vi "TouchMux-API.vi"(11 "Connection":u8) -> (0 "t3":bool, 1 "t2":bool, 2 "t1":bool, 3 "Result Value":i16)   [LabVIEW 2010]
uses:
  mindsensors-library.llb/NXTInputRefnum.ctl
  <vilib>/NXT/Block Support/HWPage.SensorType.ctl
  <vilib>/NXT/Block Support/HWPage.SensorMode.ctl
  resource/objmgr/NXTInputOutput.rc
panel:
  in  "H123":u16=800
  in  "L123":u16=724
  in  "H23":u16=723
  in  "L23":u16=659
  in  "H13":u16=658
  in  "L13":u16=600
  in  "H3":u16=599
  in  "L3":u16=500
  in  "H12":u16=460
  in  "L12":u16=370
  in  "H2":u16=290
  in  "L2":u16=210
  in  "H1":u16=160
  in  "L1":u16=60
  in  "Generic Refnum Name":T1
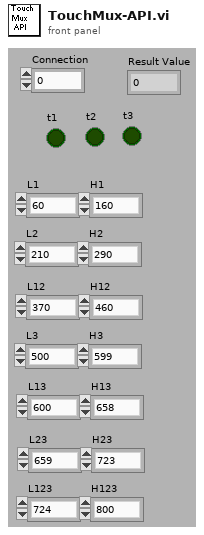
[diagram p1: front panel]
types:
  T1 = typedef "NXTInputRefnum.ctl" = refnum<k21>
  T2 = typedef "HWPage.SensorType.ctl" = u8
  T3 = typedef "HWPage.SensorMode.ctl" = u8
  T4 = typedef "NXT_InputPort.ctl" = u8
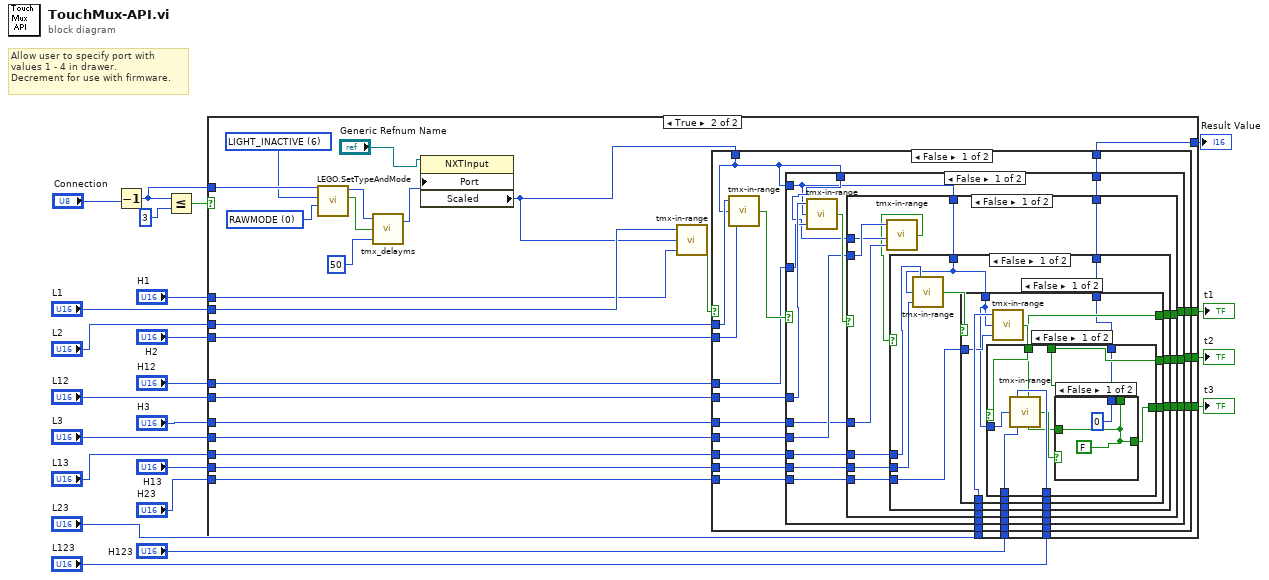
[diagram p0: block diagram]
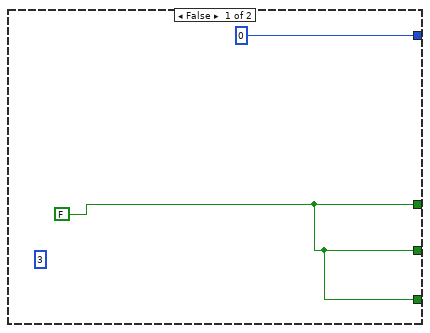
[diagram p2: hidden frame]
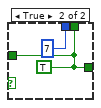
[diagram p3: hidden frame]
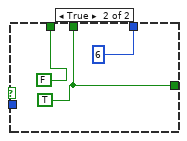
[diagram p4: hidden frame]
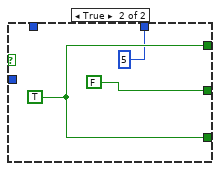
[diagram p5: hidden frame]
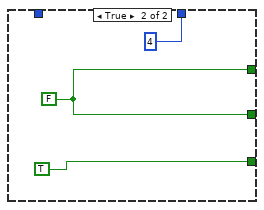
[diagram p6: hidden frame]
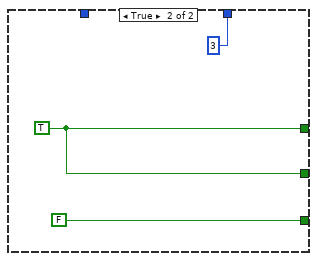
[diagram p7: hidden frame]
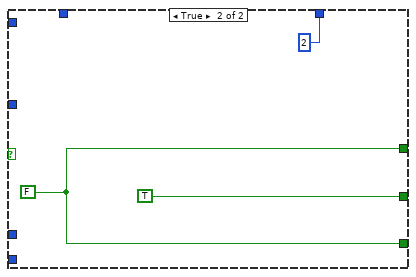
[diagram p8: hidden frame]
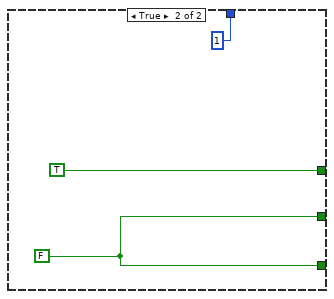
[diagram p9: hidden frame]
diagram:
  # "Allow user to specify port with\nvalues 1 - 4 in drawer. \nDecrement for use with firmware."
  n1 = Decrement(x="Connection") -> (x-1=w19:u8)
  n2 = Less Or Equal?(x=w19, y=u8 3) -> (x <= y?=w20:bool)
  n3 = case shown="True" w20 {
    tunnel: w19 -> [_ w52]
    tunnel: [u16 0 ("Raw") w25] -> w18
    tunnel: "L1" -> [_ w44]
    tunnel: "H1" -> [_ w43]
    tunnel: [w23 w41] -> w15
    tunnel: [w23 w40] -> w14
    tunnel: [w23 w39] -> w13
    tunnel: "L2" -> [_ w38]
    tunnel: "H2" -> [_ w37]
    tunnel: "L12" -> [_ w36]
    tunnel: "H12" -> [_ w35]
    tunnel: "L3" -> [_ w34]
    tunnel: "H3" -> [_ w33]
    tunnel: "L13" -> [_ w32]
    tunnel: "H13" -> [_ w31]
    tunnel: "L23" -> [_ w30]
    tunnel: "H23" -> [_ w29]
    tunnel: "H123" -> [_ w28]
    tunnel: "L123" -> [_ w27]
    frame False {
      (unwired) 3
      w23 = FALSE
    }
    frame True {
      w50 = T2 6 items=["NO_SENSOR", "SWITCH", "TEMPERATURE", "REFLECTION", "ANGLE", "LIGHT_ACTIVE", "LIGHT_INACTIVE", "SOUND_DB", "SOUND_DBA", "CUSTOM", "LOWSPEED", "LOWSPEED_9V"] ("SensorType")
      w49 = T3 0 items=["RAWMODE"=0, "BOOLEANMODE"=32, "TRANSITIONCNTMODE"=64, "PERIODCOUNTERMODE"=96, "PCTFULLSCALEMODE"=128, "CELSIUSMODE"=160, "FAHRENHEITMODE"=192, "ANGLESTEPMODE"=224] ("Sensor Mode")
      n4 = call "LEGO.SetTypeAndMode.vi"("SensorMode"=w49, "SensorType"=w50, "Input Port"=w52) -> ("Changed?"=w45:bool, "Input Port Dup"=w48:T4)  [unwired: 7 in]
      n5 = call "tmx_delayms.vi"("Delay ms"=u16 50, "Boolean"=w45, "Connection in"=w48) -> ("Connection out"=w47:u8)  [unwired: 1 in]
      n6 = property class="NXTInput"(reference="Generic Refnum Name", "Port"=w47) -> ("Scaled"=w26:i16)  [unwired: 1 in, 2 out]
      n7 = call "tmx-in-range.vi"("high"=w43, "input"=w26, "low"=w44) -> ("result"=w42:bool)  [unwired: 2 in]
      n8 = case shown="False" w42 {
        tunnel: [w67 TRUE] -> w41
        tunnel: [w66 w153] -> w40
        tunnel: [w65 w153] -> w39
        tunnel: w38 -> [w70 _]
        tunnel: w37 -> [w69 _]
        tunnel: w36 -> [w64 _]
        tunnel: w26 -> [w60 _]
        tunnel: w35 -> [w63 _]
        tunnel: w34 -> [w62 _]
        tunnel: w33 -> [w61 _]
        tunnel: w32 -> [w59 _]
        tunnel: w31 -> [w58 _]
        tunnel: w30 -> [w57 _]
        tunnel: w29 -> [w56 _]
        tunnel: w28 -> [w55 _]
        tunnel: w27 -> [w54 _]
        tunnel: [w53 1] -> w25
        frame False {
          n9 = call "tmx-in-range.vi"("high"=w69, "input"=w60, "low"=w70) -> ("result"=w68:bool)  [unwired: 2 in]
          n10 = case shown="False" w68 {
            tunnel: [w84 w150] -> w67
            tunnel: [w83 TRUE] -> w66
            tunnel: [w82 w150] -> w65
            tunnel: w64 -> [w87 _]
            tunnel: w63 -> [w86 _]
            tunnel: w62 -> [w81 _]
            tunnel: w61 -> [w80 _]
            tunnel: w60 -> [w79 _]
            tunnel: w60 -> [w78 _]
            tunnel: w59 -> [w77 _]
            tunnel: w58 -> [w76 _]
            tunnel: w57 -> [w75 _]
            tunnel: w56 -> [w74 _]
            tunnel: w55 -> [w73 _]
            tunnel: w54 -> [w72 _]
            tunnel: [w71 2] -> w53
            frame False {
              n11 = call "tmx-in-range.vi"("high"=w86, "input"=w78, "low"=w87) -> ("result"=w85:bool)  [unwired: 2 in]
              n12 = case shown="False" w85 {
                tunnel: [w97 w148] -> w84
                tunnel: [w96 w148] -> w83
                tunnel: [w98 FALSE] -> w82
                tunnel: w81 -> [w102 _]
                tunnel: w80 -> [w101 _]
                tunnel: w79 -> [w100 _]
                tunnel: w78 -> [w95 _]
                tunnel: w77 -> [w94 _]
                tunnel: w76 -> [w93 _]
                tunnel: w75 -> [w92 _]
                tunnel: w74 -> [w91 _]
                tunnel: w73 -> [w90 _]
                tunnel: w72 -> [w89 _]
                tunnel: [w88 3] -> w71
                frame False {
                  n13 = call "tmx-in-range.vi"("high"=w101, "input"=w100, "low"=w102) -> ("result"=w99:bool)  [unwired: 2 in]
                  n14 = case shown="False" w99 {
                    tunnel: [w111 TRUE] -> w98
                    tunnel: [w104 w144] -> w97
                    tunnel: [w110 w144] -> w96
                    tunnel: w95 -> [w109 _]
                    tunnel: w94 -> [w114 _]
                    tunnel: w93 -> [w113 _]
                    tunnel: w92 -> [w108 _]
                    tunnel: w91 -> [w107 _]
                    tunnel: w90 -> [w106 _]
                    tunnel: w89 -> [w105 _]
                    tunnel: [w103 4] -> w88
                    frame False {
                      n15 = call "tmx-in-range.vi"("high"=w113, "input"=w109, "low"=w114) -> ("result"=w112:bool)  [unwired: 2 in]
                      n16 = case shown="False" w112 {
                        tunnel: [w119 w142] -> w104
                        tunnel: [w121 w142] -> w111
                        tunnel: [w120 FALSE] -> w110
                        tunnel: w109 -> [w118 _]
                        tunnel: w108 -> [w124 _]
                        tunnel: w107 -> [w123 _]
                        tunnel: w106 -> [w117 _]
                        tunnel: w105 -> [w116 _]
                        tunnel: [w115 5] -> w103
                        frame False {
                          n17 = call "tmx-in-range.vi"("high"=w123, "input"=w118, "low"=w124) -> ("result"=w122:bool)  [unwired: 2 in]
                          n18 = case shown="False" w122 {
                            tunnel: [w128 w139] -> w121
                            tunnel: [w127 w139] -> w120
                            tunnel: [w126 FALSE] -> w119
                            tunnel: w118 -> [w132 _]
                            tunnel: w117 -> [w131 _]
                            tunnel: w116 -> [w130 _]
                            tunnel: [w125 6] -> w115
                            frame False {
                              n19 = call "tmx-in-range.vi"("high"=w131, "input"=w132, "low"=w130) -> ("result"=w129:bool)  [unwired: 2 in]
                              n20 = case shown="False" w129 {
                                tunnel: [w134 w136] -> w128
                                tunnel: [w134 w136] -> w127
                                tunnel: [w134 w136] -> w126
                                tunnel: [0 7] -> w125
                                frame False {
                                w134 = FALSE
                                }
                                frame True {
                                w136 = TRUE
                                }
                              }
                            }
                            frame True {
                              w139 = TRUE
                            }
                          }
                        }
                        frame True {
                          w142 = TRUE
                        }
                      }
                    }
                    frame True {
                      w144 = FALSE
                    }
                  }
                }
                frame True {
                  w148 = TRUE
                }
              }
            }
            frame True {
              w150 = FALSE
            }
          }
        }
        frame True {
          w153 = FALSE
        }
      }
    }
  }
  "Result Value" <- w18
  "t1" <- w15
  "t2" <- w14
  "t3" <- w13
